vi "Mark10 Comm.vi"(6 "Action":T2, 8 "error in (no error)":errorcluster, 10 "Write":string, 11 "VISA resource name":refnum<visa-resource-name>="COM1") -> (0 "error out":errorcluster, 1 "Flags":T1, 2 "Data Out":string, 3 "Mark-10 Ref":refnum<visa-resource-name>, 4 "NoGauge":bool, 5 "Position":dbl, 7 "Load":dbl)   [LabVIEW 2015]
uses:
  Controls/Mark10 Comm states.ctl
  <vilib>/Instr/_visa.llb/VISA Set IO Buffer Mask.ctl
  <vilib>/Instr/_visa.llb/VISA Configure Serial Port (Instr).vi
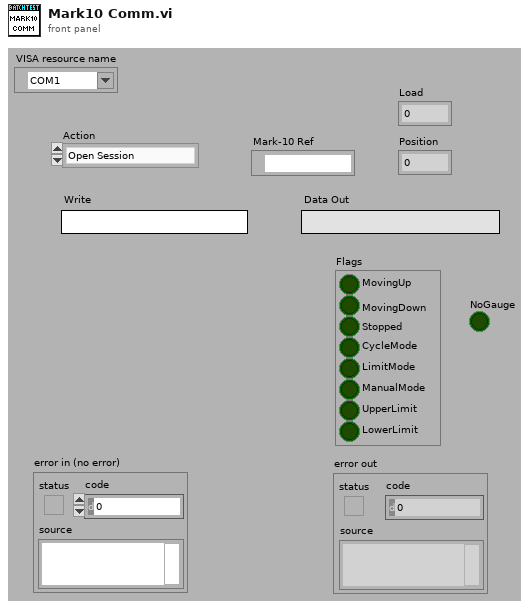
[diagram p1: front panel]
types:
  T1 = cluster{"MovingUp":bool, "MovingDown":bool, "Stopped":bool, "CycleMode":bool, "LimitMode":bool, "ManualMode":bool, "UpperLimit":bool, "LowerLimit":bool}
  T2 = typedef "Mark10 Comm states.ctl" = enum16{"Open Session", "Get Reference", "Write Data", "Read Data", "Close Session"}
  T3 = cluster{"Xceiver Ref":refnum<visa-resource-name>, "Flags":bool[], "GuagePosition":dbl, "Load":dbl, "NoGauge":bool}
  T4 = typedef "VISA Set IO Buffer Mask.ctl" = u16
  T5 = cluster{"Flags[0]":bool, "Flags[1]":bool, "Flags[2]":bool, "Flags[3]":bool, "Flags[4]":bool, "Flags[5]":bool, "Flags[6]":bool, "Flags[7]":bool}
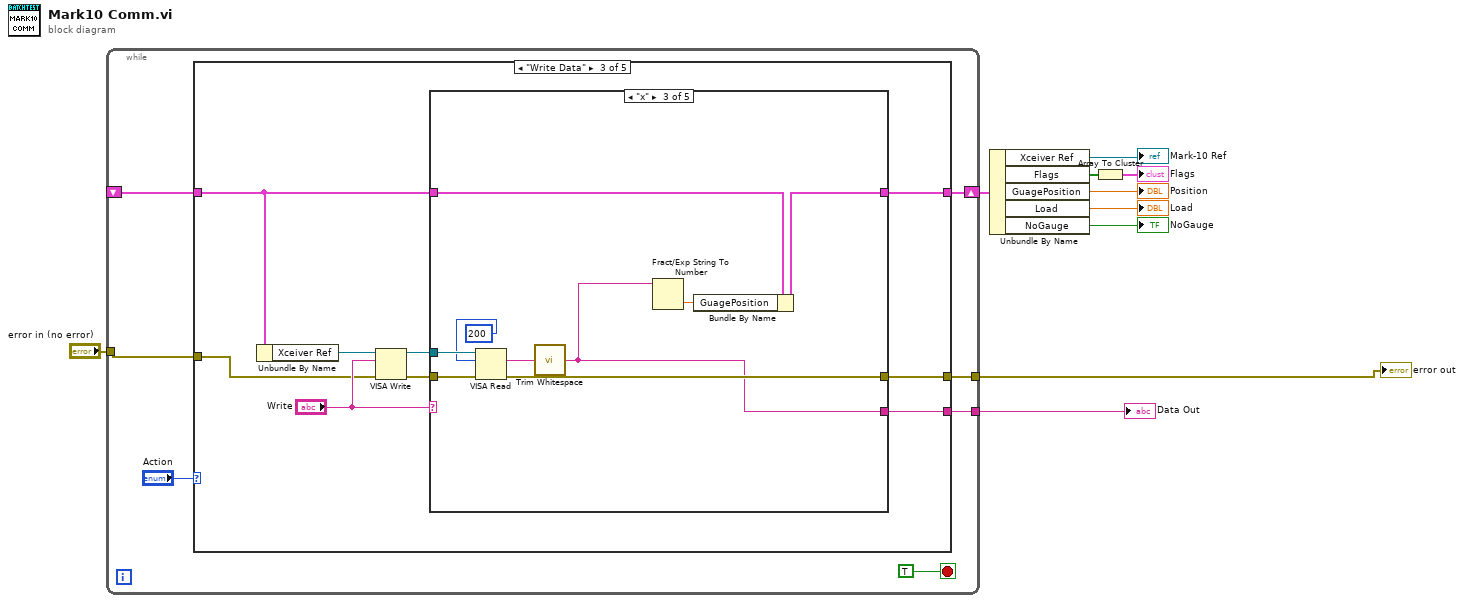
[diagram p0: block diagram]
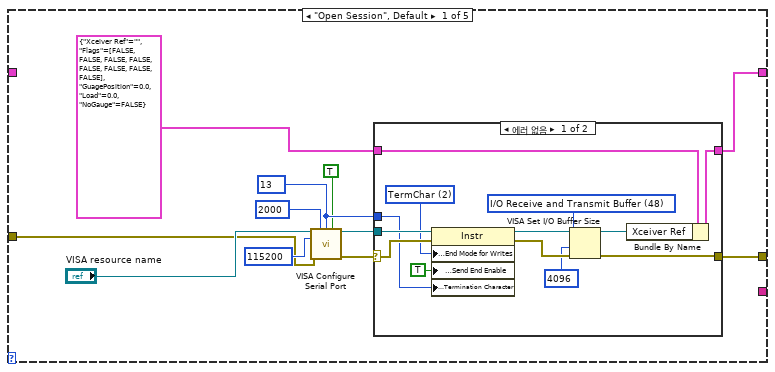
[diagram p2: hidden frame]
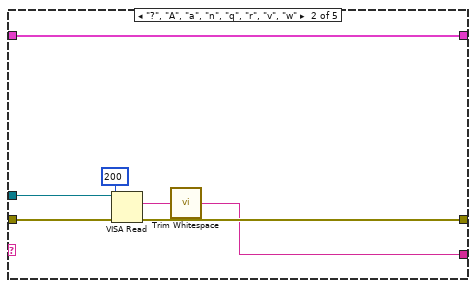
[diagram p6: hidden frame]
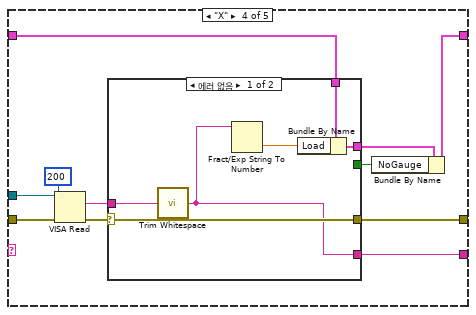
[diagram p7: hidden frame]
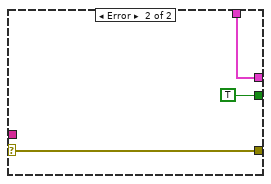
[diagram p8: hidden frame]
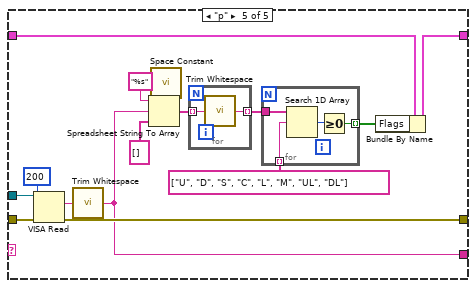
[diagram p9: hidden frame]
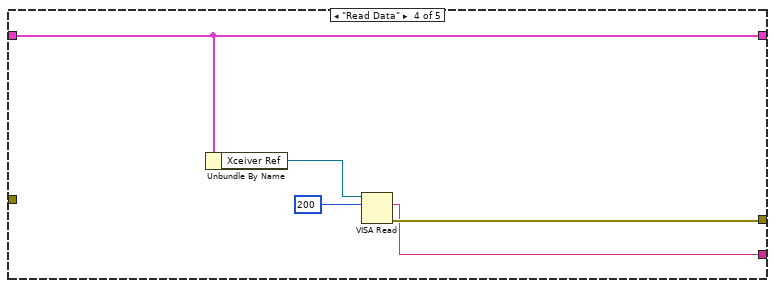
[diagram p10: hidden frame]
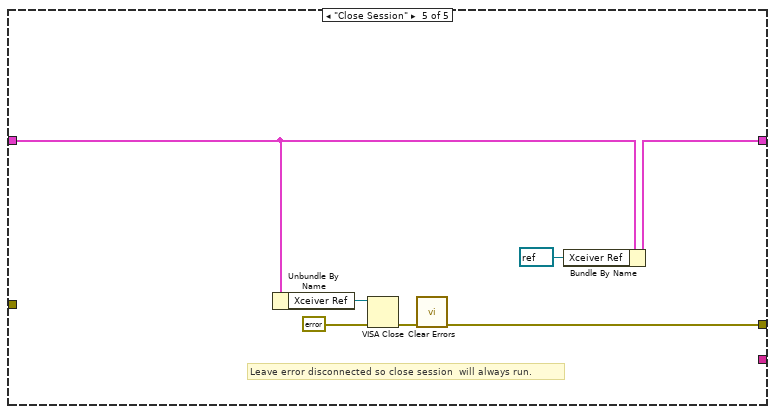
[diagram p11: hidden frame]
diagram:
  n1 = while {
    shift-right: [w15] -> w9
    shift-left: _ -> [w14]
    tunnel: [w16] -> w1
    tunnel: [w12] -> w10
    tunnel: "error in (no error)" -> [w11]
    stop <- TRUE stop-if-true
    n2 = case shown="\"Write Data\"" "Action" {
      tunnel: [w28 w44 w52 w118 w125] -> w16
      tunnel: [w27 w45 w47 w117 w123] -> w15
      tunnel: w14 -> [_ w45 w48 w117 w124]
      tunnel: [_ _ w50 w116 _] -> w12
      tunnel: w11 -> [w18 w44 w46 _ _]
      frame "Open Session", Default {
        w22 = u8 13 ("termination char\n(0xA = '\\n' = LF)")
        n3 = call-poly "VISA Configure Serial Port"("VISA resource name"="VISA resource name", "timeout (10sec)"=u32 2000, "termination char\n(0xA = '\\n' = LF)"=w22, "Enable Termination\nChar (T)"=TRUE ("Enable Termination\nChar (T)"), "baud rate (9600)"=u32 115200, "error in (no error)"=w18) -> ("VISA resource name out"=w23:refnum<visa-resource-name>, "error out"=w24:errorcluster)  [unwired: 4 in, 4 out]
        n4 = case shown="에러 없음" w24 {
          selector: w24 -> [w37 w42]
          tunnel: [w31 w42] -> w28
          tunnel: [w40 w43] -> w27
          tunnel: T3 {"Xceiver Ref"="", "Flags"=[FALSE, FALSE, FALSE, FALSE, FALSE, FALSE, FALSE, FALSE], "GuagePosition"=0.0, "Load"=0.0, "NoGauge"=FALSE} -> [w41 w43]
          tunnel: w23 -> [w38 _]
          tunnel: w22 -> [w36 _]
          frame No Error {
            w30 = T4 48 items=["I/O Receive Buffer"=16, "I/O Transmit Buffer"=32, "I/O Receive and Transmit Buffer"=48] ("Mask")
            w35 = u16 2 items=["None", "Last Bit", "TermChar", "Break"] ("Serial Settings:End Mode for Writes")
            n5 = property class="Instr"(reference=w38, error in=w37, "Serial Settings:End Mode for Writes"=w35, "Message Based Settings:Send End Enable"=TRUE, "Message Based Settings:Termination Character"=w36) -> (reference out=w34:refnum<visa-resource-name>, error out=w33:errorcluster)
            n6 = VISA Set I/O Buffer Size(VISA resource name=w34, mask (16)=w30, size (4096)=u32 4096, error in (no error)=w33) -> (VISA resource name out=w32:refnum<visa-resource-name>, error out=w31:errorcluster)
            n7 = Bundle By Name(cluster=w41, "Xceiver Ref"=w32) -> (w40:T3)
          }
          frame Error {
          }
        }
      }
      frame "Get Reference" {
      }
      frame "Write Data" {
        n8 = Unbundle By Name(w48) -> ("Xceiver Ref"=w54:refnum<visa-resource-name>)
        n9 = VISA Write(VISA resource name=w54, write buffer="Write", error in (no error)=w46) -> (VISA resource name out=w51:refnum<visa-resource-name>, error out=w53:errorcluster)  [unwired: 1 out]
        n10 = case shown="\"x\"" "Write" {
          tunnel: w53 -> [w56 w63 w72 w83 w107]
          tunnel: [w56 w62 w71 w76 w106] -> w52
          tunnel: w51 -> [_ w61 w70 w82 w105]
          tunnel: [_ w58 w66 w78 w102] -> w50
          tunnel: w48 -> [w55 w57 w67 w79 w97]
          tunnel: [w55 w57 w65 w73 w93] -> w47
          frame Default {
          }
          frame "?", "A", "a", "n", "q", "r", "v", "w" {
            n11 = VISA Read(VISA resource name=w61, byte count=u32 200, error in (no error)=w63) -> (read buffer=w59:string, error out=w62:errorcluster)  [unwired: 2 out]
            n12 = call <vilib>:"Trim Whitespace.vi"("string"=w59) -> ("trimmed string"=w58:string)  [unwired: 1 in]
          }
          frame "x" {
            n13 = VISA Read(VISA resource name=w70, byte count=u32 200, error in (no error)=w72) -> (read buffer=w68:string, error out=w71:errorcluster)  [unwired: 2 out]
            n14 = call <vilib>:"Trim Whitespace.vi"("string"=w68) -> ("trimmed string"=w66:string)  [unwired: 1 in]
            n15 = Fract/Exp String To Number(string=w66) -> (number=w64:dbl)  [unwired: 3 in, 1 out]
            n16 = Bundle By Name(cluster=w67, "GuagePosition"=w64) -> (w65:T3)
          }
          frame "X" {
            n17 = VISA Read(VISA resource name=w82, byte count=u32 200, error in (no error)=w83) -> (read buffer=w80:string, error out=w77:errorcluster)  [unwired: 2 out]
            n18 = case shown="에러 없음" w77 {
              selector: w77 -> [w86 w92]
              tunnel: w80 -> [w89 _]
              tunnel: w79 -> [w88 w90]
              tunnel: [w85 _] -> w78
              tunnel: [w86 w92] -> w76
              tunnel: [_ TRUE ("NoGauge")] -> w75
              tunnel: [w84 w90] -> w74
              frame No Error {
                n19 = call <vilib>:"Trim Whitespace.vi"("string"=w89) -> ("trimmed string"=w85:string)  [unwired: 1 in]
                n20 = Fract/Exp String To Number(string=w85) -> (number=w87:dbl)  [unwired: 3 in, 1 out]
                n21 = Bundle By Name(cluster=w88, "Load"=w87) -> (w84:T3)
              }
              frame Error {
              }
            }
            n22 = Bundle By Name(cluster=w74, "NoGauge"=w75) -> (w73:T3)
          }
          frame "p" {
            n23 = VISA Read(VISA resource name=w105, byte count=u32 200, error in (no error)=w107) -> (read buffer=w103:string, error out=w106:errorcluster)  [unwired: 2 out]
            n24 = call <vilib>:"Trim Whitespace.vi"("string"=w103) -> ("trimmed string"=w102:string)  [unwired: 1 in]
            n25 = call <vilib>:"Space Constant.vi"() -> ("String"=w101:string)
            n26 = Spreadsheet String To Array(delimiter (Tab)=w101, format string="%s", spreadsheet string=w102, array type (2D Dbl)=string[] [] ("array")) -> (array=w98:string[])
            n27 = for {
              tunnel: w98 -> [w113] mode=indexing
              tunnel: [w112] -> w96 mode=indexing
              n28 = call <vilib>:"Trim Whitespace.vi"("string"=w113) -> ("trimmed string"=w112:string)  [unwired: 1 in]
            }
            n29 = for {
              tunnel: [w110] -> w94 mode=indexing
              tunnel: w96 -> [w109]
              tunnel: string[] ["U", "D", "S", "C", "L", "M", "UL", "DL"] -> [w108] mode=indexing
              n30 = Search 1D Array(1D array=w109, element=w108) -> (index of element=w111:i32)  [unwired: 1 in]
              n31 = Greater Or Equal To 0?(x=w111) -> (x >= 0?=w110:bool)
            }
            n32 = Bundle By Name(cluster=w97, "Flags"=w94) -> (w93:T3)
          }
        }
      }
      frame "Read Data" {
        n33 = Unbundle By Name(w117) -> ("Xceiver Ref"=w115:refnum<visa-resource-name>)
        n34 = VISA Read(VISA resource name=w115, byte count=u32 200 ("Bytes To Read")) -> (read buffer=w116:string, error out=w118:errorcluster)  [unwired: 1 in, 2 out]
      }
      frame "Close Session" {
        # "Leave error disconnected so close session  will always run."
        n35 = Unbundle By Name(w124) -> ("Xceiver Ref"=w119:refnum<visa-resource-name>)
        n36 = VISA Close(VISA resource name=w119, error in (no error)=errorcluster {"status"=FALSE, "code"=0, "source"=""}) -> (error out=w121:errorcluster)
        n37 = call <vilib>:"Clear Errors.vi"("error in (no error)"=w121) -> ("error out"=w125:errorcluster)  [unwired: 5 in, 1 out]
        n38 = Bundle By Name(cluster=w124, "Xceiver Ref"=refnum<visa-resource-name> refnum ("Mark10 Ref")) -> (w123:T3)
      }
    }
  }
  "error out" <- w1
  "Data Out" <- w10
  n39 = Unbundle By Name(w9) -> ("Xceiver Ref"=→"Mark-10 Ref":refnum<visa-resource-name>, "Flags"=w7:bool[], "GuagePosition"=→"Position":dbl, "Load"=→"Load":dbl, "NoGauge"=→"NoGauge":bool)
  n40 = Array To Cluster(array=w7) -> (cluster=→"Flags":T5)
